vi "Identify Octave Version From Path.vi"(8 "error in":errorcluster, 11 "Octave path (file or bin folder)":path) -> (0 "error out":errorcluster, 1 "not identified":bool, 2 "version string":string, 3 "Octave path out":path)   [LabVIEW 2020, in "GOLPI library.lvlib"]
doc: "Tries to find Octave version string from provided Octave path."
uses:
  GOLPI library.lvlib
  <vilib>/regexp/Match Regular Expression.xnode
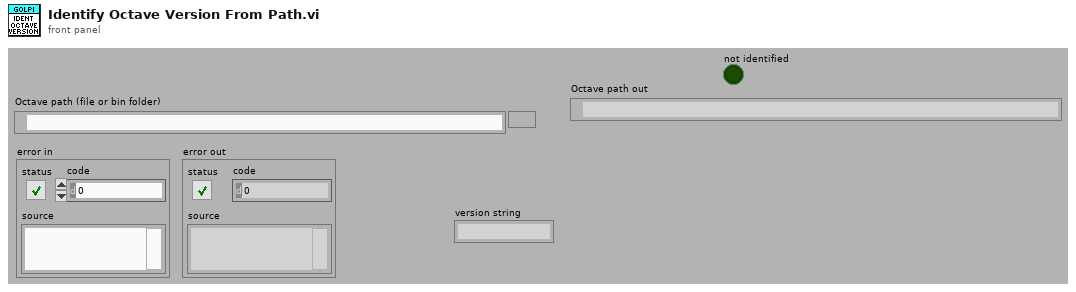
[diagram p1: front panel]
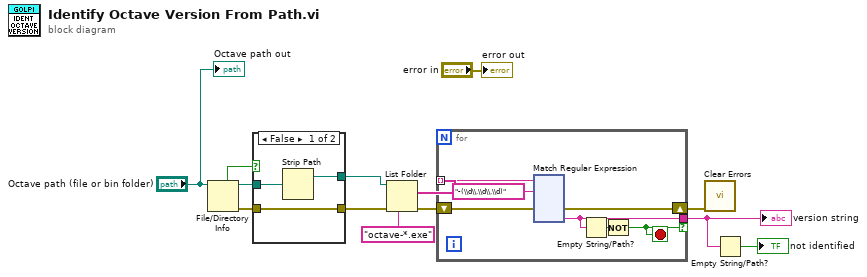
[diagram p0: block diagram]
diagram:
  n1 = File/Directory Info(path="Octave path (file or bin folder)") -> (path out=w11:path, directory=w12:bool, error out=w10:errorcluster)  [unwired: 1 in, 4 out]
  n2 = case shown="False" w12 {
    tunnel: w11 -> [w16 w18]
    tunnel: [w15 w18] -> w8
    tunnel: [w14 w17] -> w9
    tunnel: w10 -> [w14 w17]
    frame False {
      n3 = Strip Path(path=w16) -> (stripped path=w15:path)  [unwired: 1 out]
    }
    frame True {
    }
  }
  n4 = List Folder(path=w8, pattern="octave-*.exe", error in=w9) -> (filenames=w5:string[], error out=w6:errorcluster)  [unwired: 1 in, 2 out]
  n5 = for {
    tunnel: w5 -> [w24] mode=indexing
    shift-right: [w23] -> w4
    shift-left: w6 -> [w25]
    tunnel: [w20] -> w2 if=w19
    stop <- w19 stop-if-true
    n6 = xnode "Match Regular Expression"("input string"=w24, "regular expression"="-(\\d\\.\\d\\.\\d)", "error in"=w25) -> ("error out"=w23:errorcluster, "submatch 1"=w20:string)  [unwired: 3 in, 4 out]
    n7 = Empty String/Path?(string/path=w20) -> (empty?=w21:bool)
    n8 = Not(x=w21) -> (.not. x?=w19:bool)
  }
  "version string" <- w2
  n9 = call <vilib>:"Clear Errors.vi"("error in (no error)"=w4) -> ()  [unwired: 5 in, 2 out]
  n10 = Empty String/Path?(string/path=w2) -> (empty?=→"not identified":bool)
  "error out" <- "error in"
  "Octave path out" <- "Octave path (file or bin folder)"
